vi "return_axis_idx_select.vi"(7 "u(0)":sgl format="%#_13g", 8 "TsTicks":u32=1600, 11 "DAC-select":i16(ring) items=["Mod2/AO0", "Mod2/AO1", "Mod2/AO2", "Mod2/AO3", ""]) -> ()   [LabVIEW 2017]
uses:
  <vilib>/rvi/Emulation/niFpgaGetClockAttributes.vi
  <vilib>/rvi/Emulation/niFpgaSctlEmulationGetInTimedLoop.vi
  <vilib>/rvi/Emulation/niFpgaEmulationReportErrorSimple.vi
  <vilib>/rvi/Emulation/niFpgaCriticalErrorInLSC.vi
panel:
  out "Ux":sgl
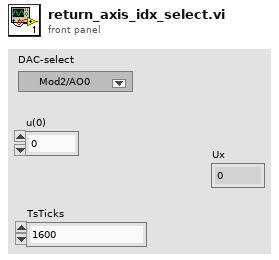
[diagram p1: front panel]
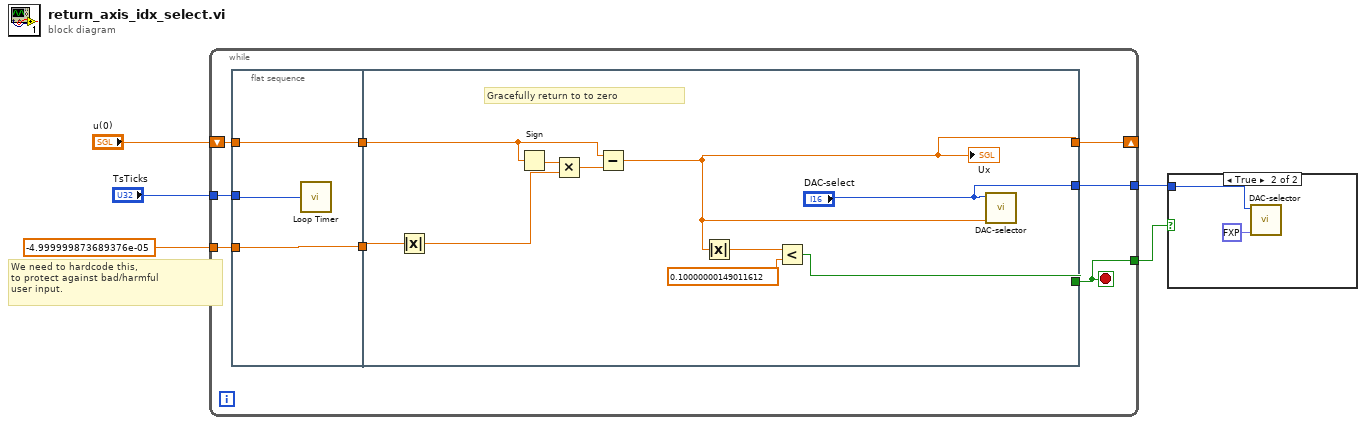
[diagram p0: block diagram]
diagram:
  # "We need to hardcode this,\nto protect against bad/harmful\nuser input."
  n1 = while {
    tunnel: sgl -5e-05 -> [w11]
    shift-right: [w10] -> _
    shift-left: "u(0)" -> [w9]
    tunnel: [w8] -> w4
    tunnel: "TsTicks" -> [w7]
    tunnel: [w6] -> w1
    stop <- w8 stop-if-true
    n2 = flat-sequence {
      tunnel: [w16] -> w13
      tunnel: w9 -> [w16]
      tunnel: [w15] -> w12
      tunnel: w11 -> [w15]
      tunnel: w7 -> [w14]
      tunnel: w13 -> [w23]
      tunnel: w12 -> [w22]
      tunnel: [w19] -> w8
      tunnel: [w18] -> w10
      tunnel: ["DAC-select"] -> w6
      frame #0 {
        n3 = call "Loop Timer"("Count(Ticks)"=w14) -> ()  [unwired: 1 out]
      }
      frame #1 {
        # "Gracefully return to to zero"
        n4 = Absolute Value(x=w22) -> (abs(x)=w21:sgl)
        n5 = Sign(1:w23) -> (0:w25:sgl)
        n6 = Multiply(x=w25, y=w21) -> (x*y=w26:sgl)
        n7 = Subtract(x=w23, y=w26) -> (x-y=w18:sgl)
        "Ux" <- w18
        n8 = Absolute Value(x=w18) -> (abs(x)=w24:sgl)
        n9 = Less?(x=w24, y=sgl 0.1) -> (x < y?=w19:bool)
        n10 = call "DAC-selector.vi"("data-in"=w18, "DAC-select"="DAC-select") -> ()  [unwired: 10 in]
      }
    }
  }
  n11 = case shown="True" w4 {
    tunnel: w1 -> [_ w28]
    frame False {
    }
    frame True {
      n12 = call "DAC-selector.vi"("data-in"=fxp<+/-,20,5> 0.0, "DAC-select"=w28) -> ()  [unwired: 10 in]
    }
  }
